vi "Set DataType.vi"(8 "error in":errorcluster, 10 "Value":refnum<class "Value.lvclass">, 11 "Object Type in":refnum<class "ARRAY.lvclass">) -> (0 "error out":errorcluster, 3 "Object Type out":refnum<class "ARRAY.lvclass">)   [LabVIEW 2024, in "EDS.lvlib" / "ARRAY.lvclass"]
uses:
  ARRAY.lvclass
  Value/Value.lvclass
  ARRAY.lvclass/ARRAY.ctl
  Object Type/Object Type Base.lvclass
  D:/git/EDS-File-Viewer/Core/Object Type/Object Type Base.lvclass
  D:/git/EDS-File-Viewer/Core/ARRAY/ARRAY.lvclass
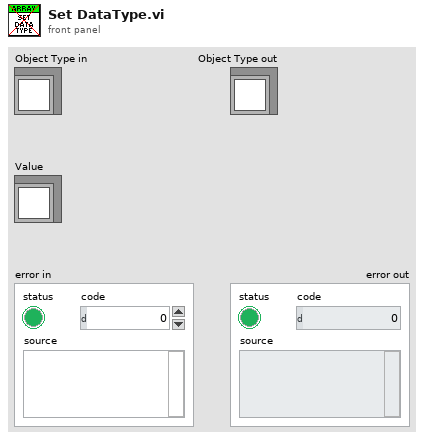
[diagram p1: front panel]
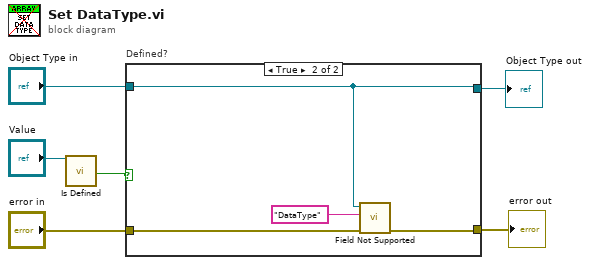
[diagram p0: block diagram]
diagram:
  n1 = call "Is Defined.vi"("Value in"="Value") -> ("Is Defined?"=w5:bool)  [unwired: 9 in, 1 out]
  n2 = case "Defined?" shown="True" w5 {
    tunnel: [w8 w11] -> w2
    tunnel: "Object Type in" -> [w7 w9]
    tunnel: [w7 w9] -> w3
    tunnel: "error in" -> [w8 w12]
    frame False {
    }
    frame True {
      n3 = call "Field Not Supported.vi"("error in"=w12, "Field name"="DataType", "Object Type in"=w9) -> ("error out"=w11:errorcluster)  [unwired: 8 in]
    }
  }
  "Object Type out" <- w3
  "error out" <- w2
